vi "PathVelocityProfile.vi"(0 "Pose":dbl[](array[numeric]), 1 "time":dbl, 3 "intervalo":dbl=0.016, 5 "estimatives":T2, 9 "Path  Smooth":dbl[][](array[numeric]), 11 "V_max":dbl format="%#_13g", 13 "Accel":dbl=10.0, 14 "DesAccel":dbl=15.0) -> (4 "Time X":dbl[](array[numeric]), 6 "Velocities X":dbl[](array[numeric]), 8 "Time Y":dbl[](array[numeric]), 10 "Velocities Y":dbl[](array[numeric]))   [LabVIEW 2018]
uses:
  Controle/VelocityProfileState.ctl
  <vilib>/Analysis/_algsub.llb/Real Vector Norm.vi
  <vilib>/Analysis/coordinate.llb/Wrap Angle (scalar).vi
  <vilib>/Analysis/NI_AAL_Angle.lvlib
  <vilib>/Analysis/NI_AALPro.lvlib
panel:
  out "VelocityProfile Y":T1[](array[typedef])
  out "VelocityProfile X":T1[](array[typedef])
  out "Velocity Profile Y":cluster{dbl[], dbl[]}[](graph)
  out "Velocity Profile X":cluster{dbl[], dbl[]}[](graph)
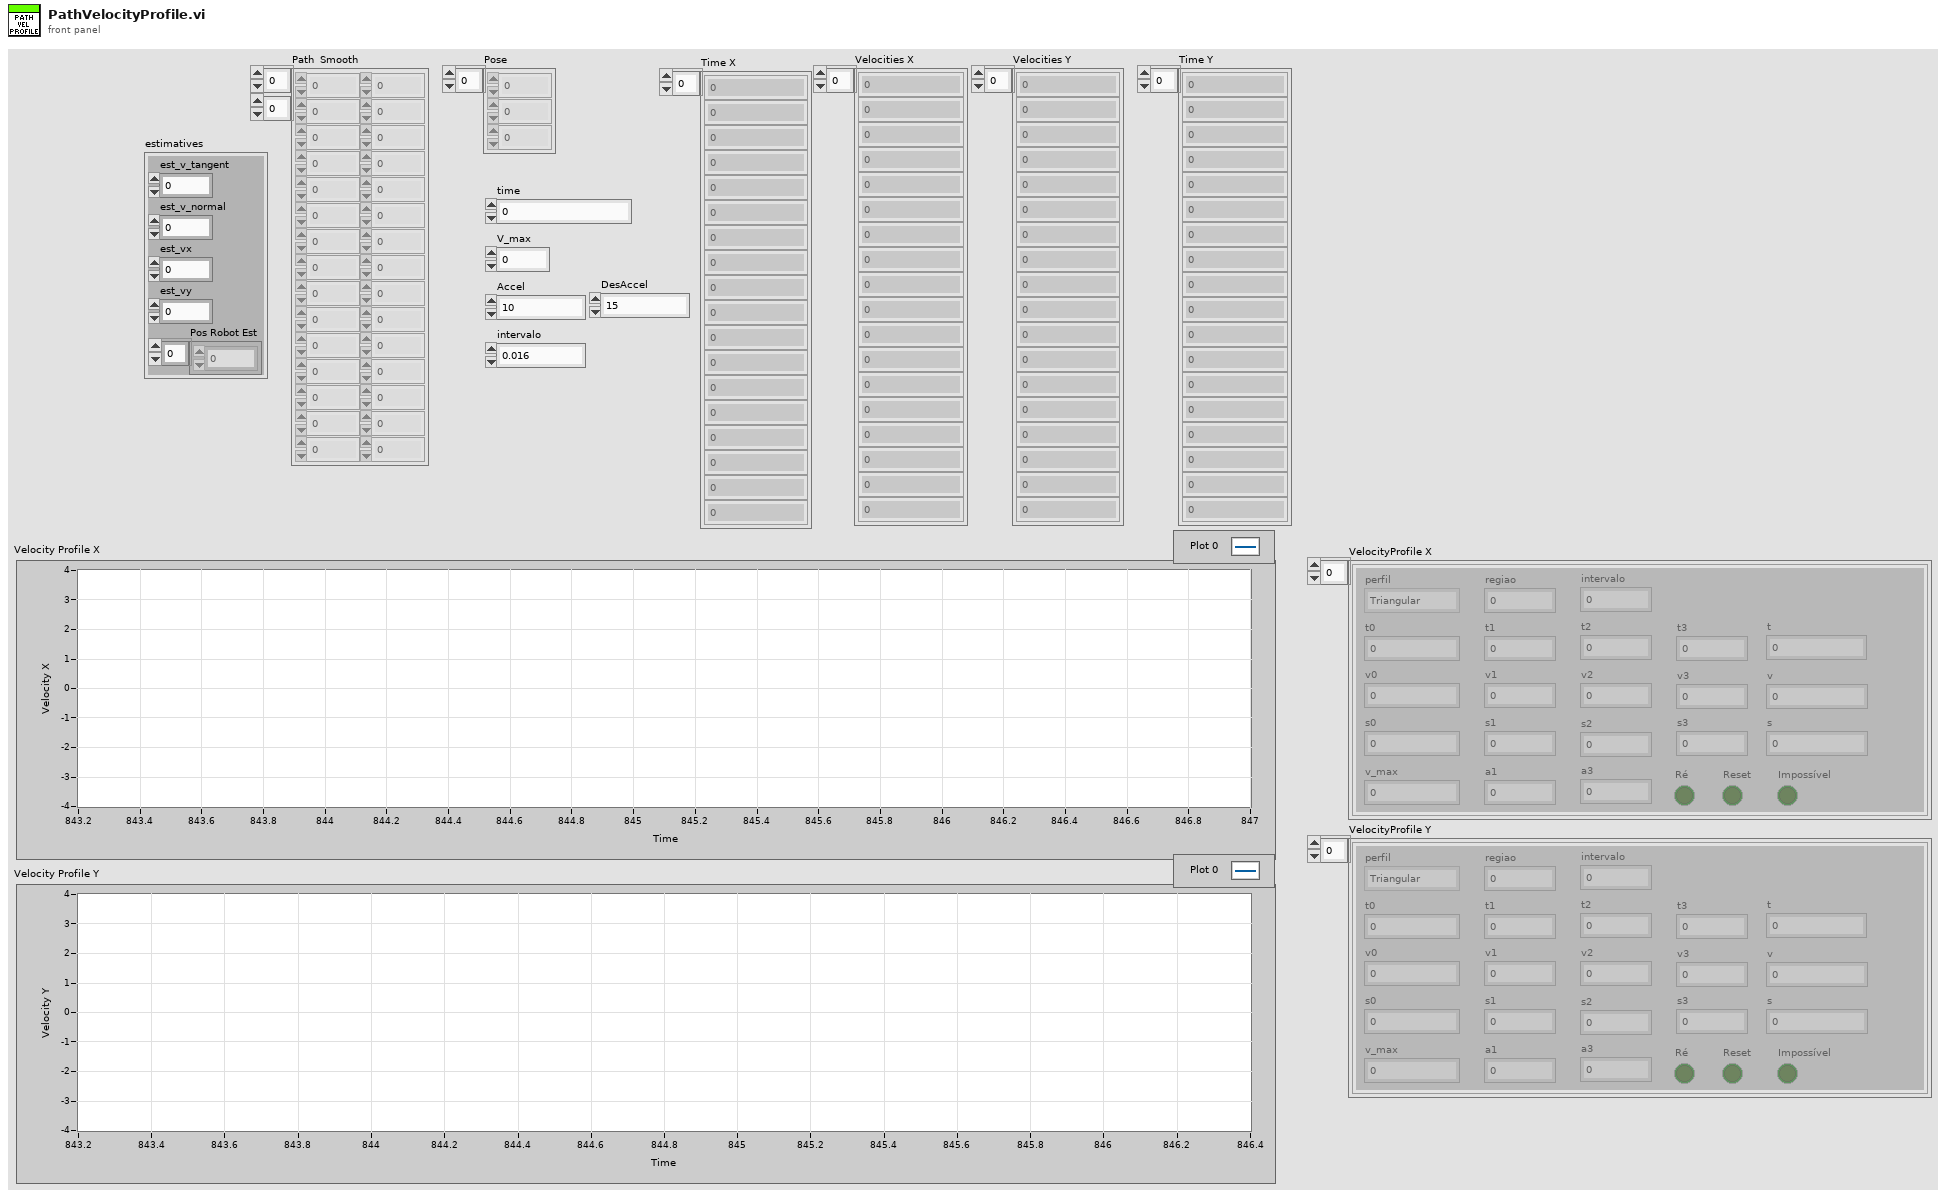
[diagram p1: front panel]
types:
  T1 = typedef "VelocityProfileState.ctl" = cluster{"t0":dbl, "t1":dbl, "t2":dbl, "t3":dbl, "v0":dbl, "v_max":dbl, "v3":dbl, "v2":dbl, "v1":dbl, "perfil":enum16{"Triangular", "Trapezoidal"}, "regiao":i32, "s0":dbl, "s1":dbl, "s2":dbl, "v":dbl, "t":dbl, "a1":dbl, "s3":dbl, "Reset":bool, "s":dbl, "a3":dbl, "Ré":bool, "Impossível":bool, "intervalo":dbl}
  T2 = cluster{"est_v_tangent":dbl, "est_v_normal":dbl, "est_vx":dbl, "est_vy":dbl, "Pos Robot Est":dbl[]}
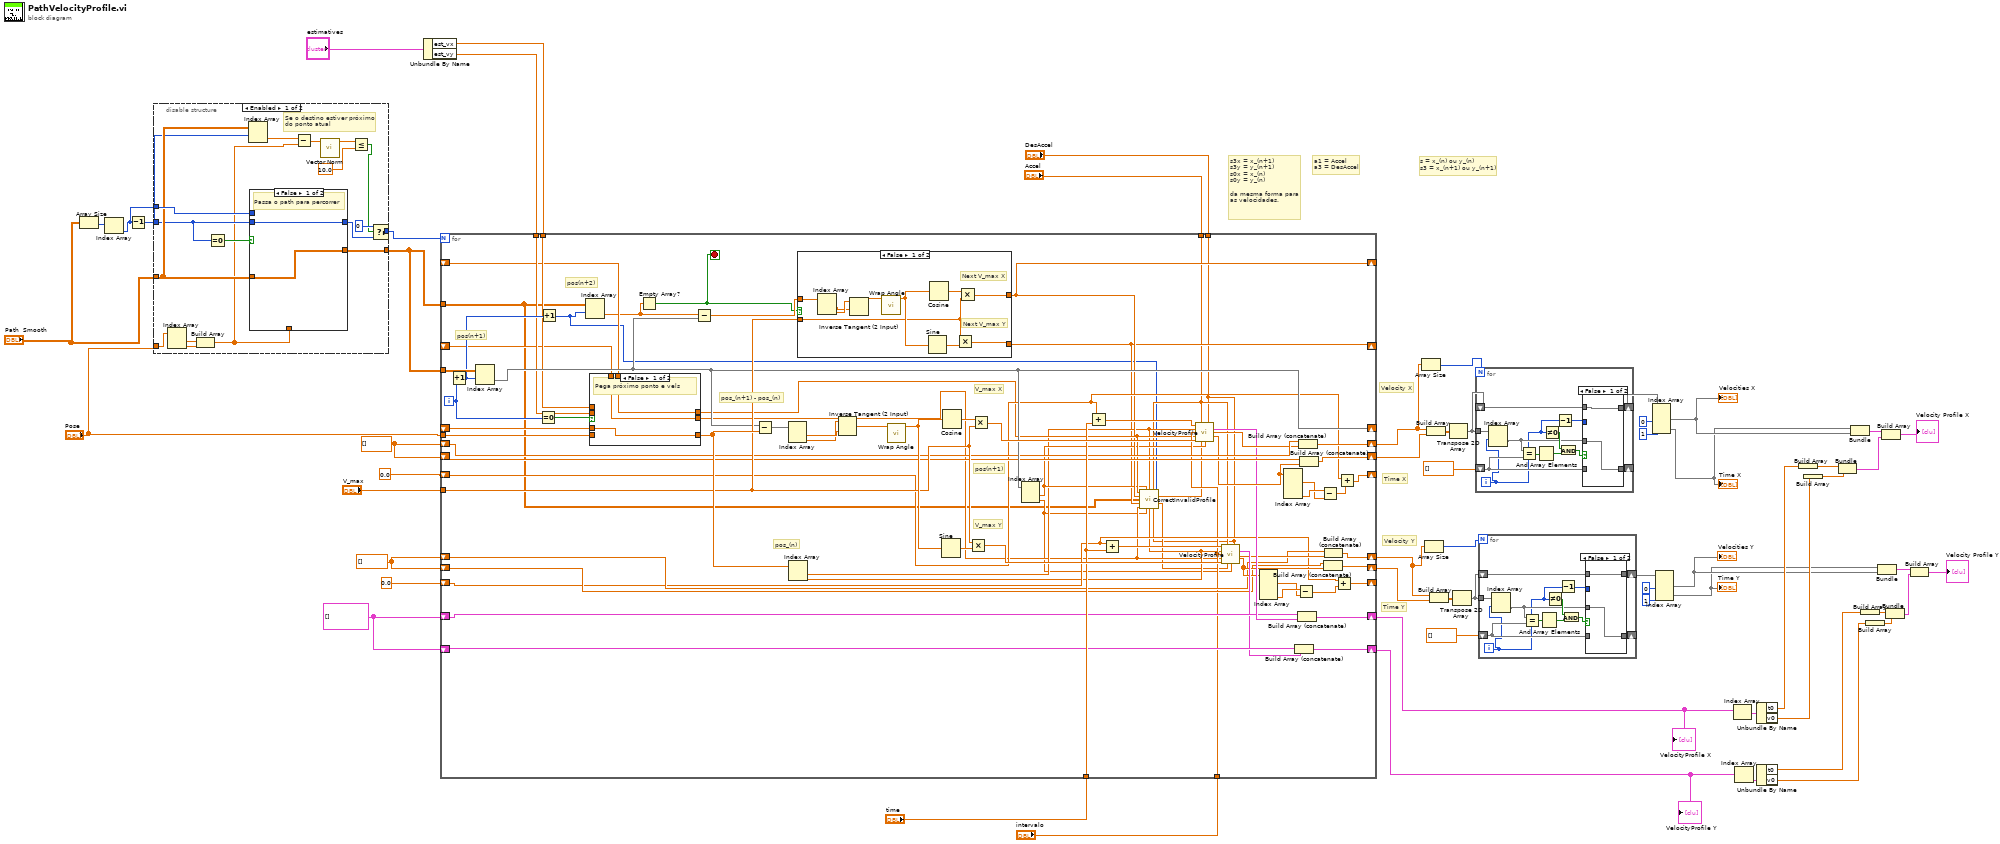
[diagram p0: block diagram]
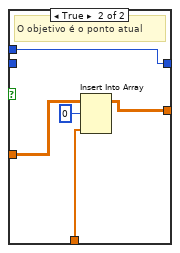
[diagram p2: hidden frame]
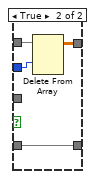
[diagram p4: hidden frame]
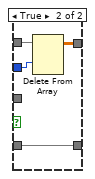
[diagram p5: hidden frame]
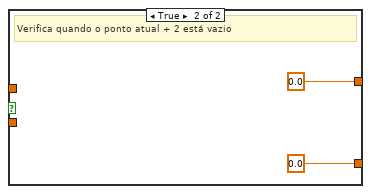
[diagram p6: hidden frame]
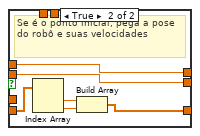
[diagram p7: hidden frame]
diagram:
  w48 = T1[] []
  w50 = dbl[] []
  w49 = dbl[] []
  # "s = x_(n) ou y_(n)\ns3 = x_(n+1) ou y_(n+1)"
  # "a1 = Accel\na3 = DesAccel"
  # "s3x = x_(n+1)\ns3y = y_(n+1)\ns0x = x_(n)\ns0y = y_(n)\n\nda mesma forma para\nas velocidades."
  # "Time X"
  # "Time Y"
  # "Velocity Y"
  # "Velocity X"
  n1 = Array Size(array="Path  Smooth") -> (size(s)=w53:i32[])
  n2 = Index Array(array=w53) -> (element=w6:i32)  [unwired: 1 in]
  n3 = Decrement(x=w6) -> (x-1=w3:i32)
  n4 = disable-structure shown="Enabled" {
    disable-tunnel: [w77 w85] -> w2
    disable-tunnel: w6 -> [w75 _]
    disable-tunnel: "Pose" -> [w74 _]
    disable-tunnel: [w71 w86] -> w1
    disable-tunnel: "Path  Smooth" -> [w68 w85]
    disable-tunnel: w3 -> [w67 w86]
    frame Enabled {
      # "Se o destino estiver próximo\ndo ponto atual"
      n5 = Index Array(array=w74) -> (element #1=w73:dbl, element #2=w72:dbl)  [unwired: 2 in]
      n6 = Build Array(w73, w72) -> (w65:dbl[])
      n7 = Equal To 0?(x=w67) -> (x = 0?=w76:bool)
      n8 = Index Array(array=w68, index (row)=w67) -> (element=w66:dbl[])  [unwired: 1 in]
      n9 = case shown="False" w76 {
        tunnel: [w78 w80] -> w77
        tunnel: w68 -> [w78 w82]
        tunnel: [w79 w84] -> w70
        tunnel: w67 -> [w79 _]
        tunnel: w75 -> [_ w84]
        tunnel: w65 -> [_ w83]
        frame False {
          # "Passa o path para percorrer"
        }
        frame True {
          # "O objetivo é o ponto atual"
          n10 = Insert Into Array(array=w82, index (row)=0, new element=w83) -> (w80:dbl[][])  [unwired: 1 in]
        }
      }
      n11 = Subtract(x=w66, y=w65) -> (x-y=w64:dbl[])
      n12 = call-poly <vilib>:"Vector Norm.vi"("Input Vector"=w64) -> ("norm"=w63:dbl)  [unwired: 9 in, 1 out]
      n13 = Less Or Equal?(x=w63, y=10.0) -> (x <= y?=w61:bool)
      n14 = Select(t=0, s=w61, f=w70) -> (s? t:f=w71:i32)
    }
    frame Disabled {
    }
  }
  n15 = Unbundle By Name("estimatives") -> ("est_vx"=w52:dbl, "est_vy"=w51:dbl)
  n16 = for {
    N: w1 -> [_]
    tunnel: w2 -> [w138]
    tunnel: "Pose" -> [w156]
    shift-right: [w139] -> _
    shift-left: _ -> [w155]
    tunnel: "V_max" -> [w143]
    tunnel: "Accel" -> [w92]
    tunnel: "DesAccel" -> [w91]
    tunnel: w2 -> [w88]
    shift-right: [w107] -> _
    shift-left: 0.0 ("t3") -> [w109]
    shift-right: [w105] -> _
    shift-left: 0.0 ("t3") -> [w104]
    tunnel: "time" -> [w141]
    shift-right: [w132] -> w27
    shift-left: w49 -> [w137]
    shift-right: [w135] -> w30
    shift-left: w49 -> [w136]
    shift-right: [w113] -> w9
    shift-left: w50 -> [w111]
    shift-right: [w112] -> w10
    shift-left: w50 -> [w110]
    tunnel: w52 -> [w129]
    tunnel: w51 -> [w128]
    shift-right: [w101] -> _
    shift-left: _ -> [w127]
    shift-right: [w95] -> _
    shift-left: _ -> [w126]
    shift-right: [w118] -> w46
    shift-left: w48 -> [w121]
    shift-right: [w117] -> w45
    shift-left: w48 -> [w120]
    tunnel: "intervalo" -> [w103]
    i -> [w89]
    stop <- w130 stop-if-true
    # "pos(n+2)"
    # "pos(n+1)"
    # "pos(n+1)"
    # "pos_(n)"
    # "pos_(n+1) - pos_(n)"
    # "V_max Y"
    # "V_max X"
    n17 = Increment(x=w89) -> (x+1=w134:i32)
    n18 = Index Array(array=w138, index (row)=w134) -> (element=w139:dbl[])  [unwired: 1 in]
    n19 = Equal To 0?(x=w89) -> (x = 0?=w157:bool)
    n20 = Increment(x=w134) -> (x+1=w87:i32)
    n21 = Index Array(array=w88, index (row)=w87) -> (element=w90:dbl[])  [unwired: 1 in]
    n22 = case shown="False" w157 {
      tunnel: w156 -> [_ w178]
      tunnel: [w172 w175] -> w147
      tunnel: w155 -> [w172 _]
      tunnel: w129 -> [_ w174]
      tunnel: w128 -> [_ w173]
      tunnel: [w170 w174] -> w102
      tunnel: [w171 w173] -> w97
      tunnel: w127 -> [w170 _]
      tunnel: w126 -> [w171 _]
      frame False {
        # "Pega próximo ponto e vels"
      }
      frame True {
        # "Se é o ponto inicial, pega a pose\ndo robô e suas velocidades"
        n23 = Index Array(array=w178) -> (element #1=w177:dbl, element #2=w176:dbl)  [unwired: 2 in]
        n24 = Build Array(w177, w176) -> (w175:dbl[])
      }
    }
    n25 = Empty Array?(array=w90) -> (empty?=w130:bool)
    n26 = Subtract(x=w90, y=w139) -> (x-y=w144:dbl[])
    n27 = Subtract(x=w139, y=w147) -> (x-y=w153:dbl[])
    n28 = Index Array(array=w153) -> (element #1=w154:dbl, element #2=w152:dbl)  [unwired: 2 in]
    n29 = Index Array(array=w147) -> (element #1=w99:dbl, element #2=w98:dbl)  [unwired: 2 in]
    n30 = case shown="False" w130 {
      tunnel: w144 -> [w162 _]
      tunnel: w143 -> [w160 _]
      tunnel: [w159 0.0] -> w101
      tunnel: [w158 0.0] -> w95
      frame False {
        # "Next V_max Y"
        # "Next V_max X"
        n31 = Index Array(array=w162) -> (element #1=w161:dbl, element #2=w163:dbl)  [unwired: 2 in]
        n32 = Inverse Tangent (2 Input)(1:w161, 2:w163) -> (0:w164:dbl)
        n33 = call-poly <vilib>:"Wrap Angle.vi"("angle in"=w164) -> ("angle out"=w165:dbl)  [unwired: 9 in, 1 out]
        n34 = Sine(x=w165) -> (sin(x)=w167:dbl)
        n35 = Cosine(x=w165) -> (cos(x)=w166:dbl)
        n36 = Multiply(x=w160, y=w167) -> (x*y=w158:dbl)
        n37 = Multiply(x=w166, y=w160) -> (x*y=w159:dbl)
      }
      frame True {
        # "Verifica quando o ponto atual + 2 está vazio"
      }
    }
    n38 = Inverse Tangent (2 Input)(1:w154, 2:w152) -> (0:w151:dbl)
    n39 = call-poly <vilib>:"Wrap Angle.vi"("angle in"=w151) -> ("angle out"=w150:dbl)  [unwired: 9 in, 1 out]
    n40 = Sine(x=w150) -> (sin(x)=w148:dbl)
    n41 = Cosine(x=w150) -> (cos(x)=w149:dbl)
    n42 = Multiply(x=w143, y=w148) -> (x*y=w145:dbl)
    n43 = Multiply(x=w149, y=w143) -> (x*y=w146:dbl)
    n44 = Index Array(array=w139) -> (element #1=w100:dbl, element #2=w96:dbl)  [unwired: 2 in]
    n45 = Add(x=w109, y=w141) -> (x+y=w142:dbl)
    n46 = Add(x=w104, y=w141) -> (x+y=w140:dbl)
    n47 = call "CorrectInvalidProfile.vi"("v0x"=w102, "s3x"=w100, "s0x"=w99, "a1"=w92, "index"=w87, "v3x"=w101, "Path  Smooth"=w88, "v3y"=w95, "v0y"=w97, "s3y"=w96, "s0y"=w98, "a3"=w91) -> ("New v3x"=w93:dbl, "New v3y"=w94:dbl)  [unwired: 2 in]
    n48 = call "VelocityProfile.vi"("t"=w142, "a1"=w92, "a3"=w91, "s"=w99, "intervalo"=w103, "v_est"=w102, "v_max"=w146, "v3"=w93, "s3"=w100) -> ("VelocityProfileState Out"=w122:T1, "Velocities"=w133:dbl[], "Time"=w131:dbl[])  [unwired: 3 in, 1 out]
    n49 = call "VelocityProfile.vi"("t"=w140, "a1"=w92, "a3"=w91, "s"=w98, "intervalo"=w103, "v_est"=w97, "v_max"=w145, "v3"=w94, "s3"=w96) -> ("VelocityProfileState Out"=w119:T1, "Velocities"=w116:dbl[], "Time"=w114:dbl[])  [unwired: 3 in, 1 out]
    n50 = Index Array(array=w114) -> (element #1=w124:dbl, element #4=w125:dbl)  [unwired: 4 in, 2 out]
    n51 = Index Array(array=w131) -> (element #1=w115:dbl, element #4=w123:dbl)  [unwired: 4 in, 2 out]
    n52 = Build Array (concatenate)(w120, w119) -> (w117:T1[])
    n53 = Subtract(x=w125, y=w124) -> (x-y=w106:dbl)
    n54 = Build Array (concatenate)(w121, w122) -> (w118:T1[])
    n55 = Build Array (concatenate)(w137, w133) -> (w132:dbl[])
    n56 = Build Array (concatenate)(w136, w131) -> (w135:dbl[])
    n57 = Subtract(x=w123, y=w115) -> (x-y=w108:dbl)
    n58 = Build Array (concatenate)(w110, w114) -> (w112:dbl[])
    n59 = Build Array (concatenate)(w111, w116) -> (w113:dbl[])
    n60 = Add(x=w104, y=w106) -> (x+y=w105:dbl)
    n61 = Add(x=w109, y=w108) -> (x+y=w107:dbl)
  }
  "VelocityProfile X" <- w46
  "VelocityProfile Y" <- w45
  n62 = Array Size(array=w27) -> (size(s)=w24:i32)
  n63 = Array Size(array=w9) -> (size(s)=w13:i32)
  n64 = Build Array(w27, w30) -> (w23:dbl[][])
  n65 = Build Array(w9, w10) -> (w14:dbl[][])
  n66 = Transpose 2D Array(2D array=w23) -> (transposed array=w22:dbl[][])
  n67 = Transpose 2D Array(2D array=w14) -> (transposed array=w15:dbl[][])
  n68 = for {
    N: w24 -> [_]
    tunnel: w22 -> [w182]
    shift-right: [w190] -> _
    shift-left: dbl[] [] -> [w189]
    shift-right: [w183] -> w25
    shift-left: w22 -> [w184]
    i -> [w179]
    n69 = Index Array(array=w182, index (row)=w179) -> (element=w181:dbl[])  [unwired: 1 in]
    n70 = Equal?(x=w181, y=w189) -> (x = y?=w188:bool[])
    n71 = And Array Elements(Boolean array=w188) -> (logical AND=w187:bool)
    n72 = Not Equal To 0?(x=w179) -> (x != 0?=w186:bool)
    n73 = Decrement(x=w179) -> (x-1=w180:i32)
    n74 = And(x=w186, y=w187) -> (x .and. y?=w185:bool)
    n75 = case shown="False" w185 {
      tunnel: w181 -> [w192 _]
      tunnel: [w192 w196] -> w190
      tunnel: w189 -> [_ w196]
      tunnel: w184 -> [w191 w195]
      tunnel: [w191 w194] -> w183
      tunnel: w180 -> [_ w193]
      frame False {
      }
      frame True {
        n76 = Delete From Array(array=w195, index (row)=w193) -> (array with subset deleted=w194:dbl[][])  [unwired: 2 in, 1 out]
      }
    }
  }
  n77 = for {
    N: w13 -> [_]
    tunnel: w15 -> [w200]
    shift-right: [w208] -> _
    shift-left: dbl[] [] -> [w207]
    shift-right: [w201] -> w12
    shift-left: w15 -> [w202]
    i -> [w197]
    n78 = Index Array(array=w200, index (row)=w197) -> (element=w199:dbl[])  [unwired: 1 in]
    n79 = Equal?(x=w199, y=w207) -> (x = y?=w206:bool[])
    n80 = And Array Elements(Boolean array=w206) -> (logical AND=w205:bool)
    n81 = Not Equal To 0?(x=w197) -> (x != 0?=w204:bool)
    n82 = Decrement(x=w197) -> (x-1=w198:i32)
    n83 = And(x=w204, y=w205) -> (x .and. y?=w203:bool)
    n84 = case shown="False" w203 {
      tunnel: w199 -> [w210 _]
      tunnel: [w210 w214] -> w208
      tunnel: w207 -> [_ w214]
      tunnel: w202 -> [w209 w213]
      tunnel: [w209 w212] -> w201
      tunnel: w198 -> [_ w211]
      frame False {
      }
      frame True {
        n85 = Delete From Array(array=w213, index (row)=w211) -> (array with subset deleted=w212:dbl[][])  [unwired: 2 in, 1 out]
      }
    }
  }
  n86 = Index Array(array=w25, index (col) #1=0 ("disabled index (col)"), index (col) #2=1 ("index (col)")) -> (element #1=w29:dbl[], element #2=w28:dbl[])  [unwired: 2 in]
  "Velocities X" <- w29
  "Time X" <- w28
  n87 = Index Array(array=w12, index (col) #1=0 ("disabled index (col)"), index (col) #2=1 ("index (col)")) -> (element #1=w8:dbl[], element #2=w7:dbl[])  [unwired: 2 in]
  "Velocities Y" <- w8
  "Time Y" <- w7
  n88 = Index Array(array=w46) -> (element=w44:T1)  [unwired: 1 in]
  n89 = Index Array(array=w45) -> (element=w43:T1)  [unwired: 1 in]
  n90 = Unbundle By Name(w44) -> ("t0"=w36:dbl, "v0"=w35:dbl)
  n91 = Unbundle By Name(w43) -> ("t0"=w32:dbl, "v0"=w31:dbl)
  n92 = Build Array(w36) -> (w37:dbl[])
  n93 = Build Array(w35) -> (w38:dbl[])
  n94 = Bundle(w37, w38) -> (w18:cluster{dbl[], dbl[]})  [unwired: 1 in]
  n95 = Bundle(w28, w29) -> (w42:cluster{dbl[], dbl[]})  [unwired: 1 in]
  n96 = Build Array(w32) -> (w33:dbl[])
  n97 = Build Array(w31) -> (w34:dbl[])
  n98 = Bundle(w7, w8) -> (w40:cluster{dbl[], dbl[]})  [unwired: 1 in]
  n99 = Build Array(w42, w18) -> (→"Velocity Profile X":cluster{dbl[], dbl[]}[])
  n100 = Bundle(w33, w34) -> (w19:cluster{dbl[], dbl[]})  [unwired: 1 in]
  n101 = Build Array(w40, w19) -> (→"Velocity Profile Y":cluster{dbl[], dbl[]}[])
